vi "WebSocket Conection Check.vi"(8 "error in":errorcluster, 11 "Connection In":refnum<k5>) -> (0 "error out":errorcluster, 3 "Connection Out":refnum<k5>)   [LabVIEW 2018]
uses:
  Data Def/WebSocket Manerger Method.ctl
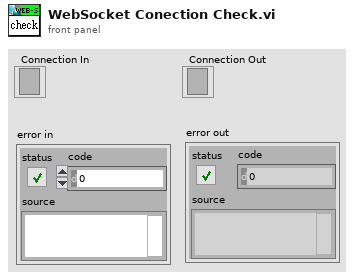
[diagram p1: front panel]
types:
  T1 = typedef "WebSocket Manerger Method.ctl" = enum16{"Initialize", "Add Connection", "Get Connections", "Close Connection", "Close All"}
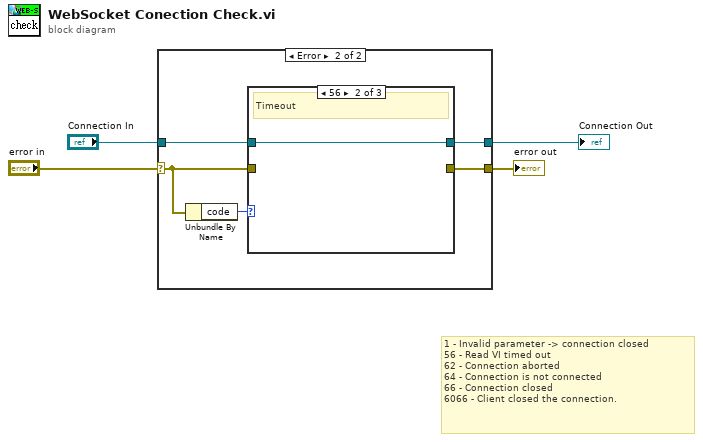
[diagram p0: block diagram]
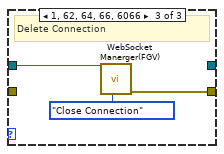
[diagram p4: hidden frame]
diagram:
  # "1 - Invalid parameter -> connection closed\n56 - Read VI timed out\n62 - Connection aborted\n64 - Connection is not connected\n66 - Connection closed\n6066 - Client closed the connection."
  n1 = case shown="Error" "error in" {
    selector: "error in" -> [w6 w7]
    tunnel: [w6 w8] -> w3
    tunnel: "Connection In" -> [w5 w10]
    tunnel: [w5 w9] -> w1
    frame No Error {
    }
    frame Error {
      n2 = Unbundle By Name(w7) -> ("code"=w11:i32)
      n3 = case shown="56" w11 {
        tunnel: w10 -> [w13 w14 w16]
        tunnel: [w13 w14 _] -> w9
        tunnel: [w12 _ w15] -> w8
        tunnel: w7 -> [w12 _ _]
        frame 0, Default {
          # "Exception"
        }
        frame 56 {
          # "Timeout"
        }
        frame 1, 62, 64, 66, 6066 {
          # "Delete Connection"
          n4 = call "WebSocket Manerger(FGV).vi"("WebSocket Manerger Method"=WebSocket_Manerger_Method."Close Connection", "connection In"=w16) -> ("error out"=w15:errorcluster)  [unwired: 8 in, 1 out]
        }
      }
    }
  }
  "error out" <- w3
  "Connection Out" <- w1
